vi "Definition.vi"(11 "Long Class Name Entity Example":refnum<class "Long Class Name Entity Example.lvclass">) -> (2 "Entity Definition":refnum<class "Type.lvclass">[](array[class]))   [LabVIEW 2020, in "Conditum-Example.lvlib" / "Long Class Name Entity Example.lvclass"]
uses:
  Long Class Name Entity Example.lvclass
  Conditum/Columns/Type/Type.lvclass
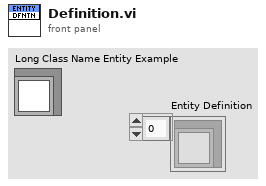
[diagram p1: front panel]
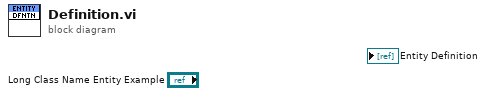
[diagram p0: block diagram]
diagram:
